vi "_kafkaEventsToWaveform - Copy.vi"(8 "error":errorcluster, 10 "Waveform Datatype":variant, 11 "Kafka Events":T1[](array[typedef])) -> (0 "error out":errorcluster, 3 "Waveforms":waveform(dbl)[](array[waveform]), 5 "Names":string[][](array[string]), 7 "Values":variant[][](array[variant]))   [LabVIEW 2019]
uses:
  KafkaLVLib/API/KafkaConsumerEvent.ctl
  b523245a-1091-4a37-a3a5-079169cc6668.vi
  54bb518a-e9be-4d14-b53e-b2dc3388e6d5.vi
  fe8c1a35-af5e-47a5-bbcb-22ec2aeec76b.vi
  <vilib>/JDP Science/JSONtext/String Subset.vi
  <vilib>/JDP Science/JSONtext/Parsing/Parse Full Path or Item Name.vi
  <vilib>/JDP Science/JSONtext/Next JSON Value.vi
  <vilib>/JDP Science/JSONtext/support/Error Cluster From Code.vi
  <vilib>/JDP Science/JSONtext/Offset/Find Item Locations by Path.vi
  <vilib>/JDP Science/JSONtext/JSON text to Variant.vi
  <vilib>/JDP Science/JSONtext/JSONtext.lvlib
panel:
  out "Measured Data":waveform(dbl)[](graph)
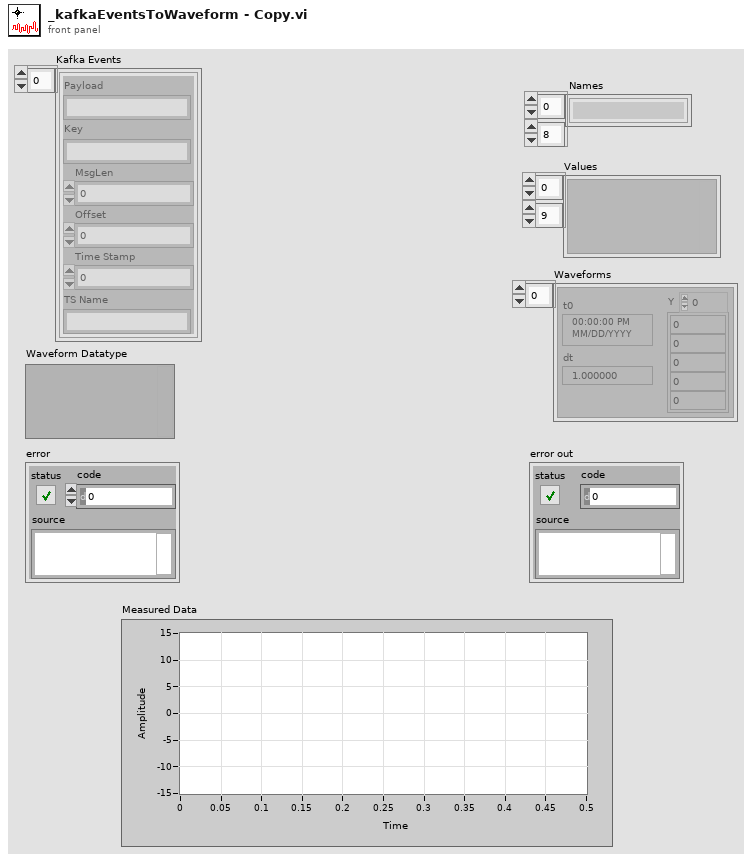
[diagram p1: front panel]
types:
  T1 = typedef "KafkaConsumerEvent.ctl" = cluster{"Payload":string, "Key":string, "MsgLen":u64, "Offset":i64, "Time Stamp":i64, "TS Name":string}
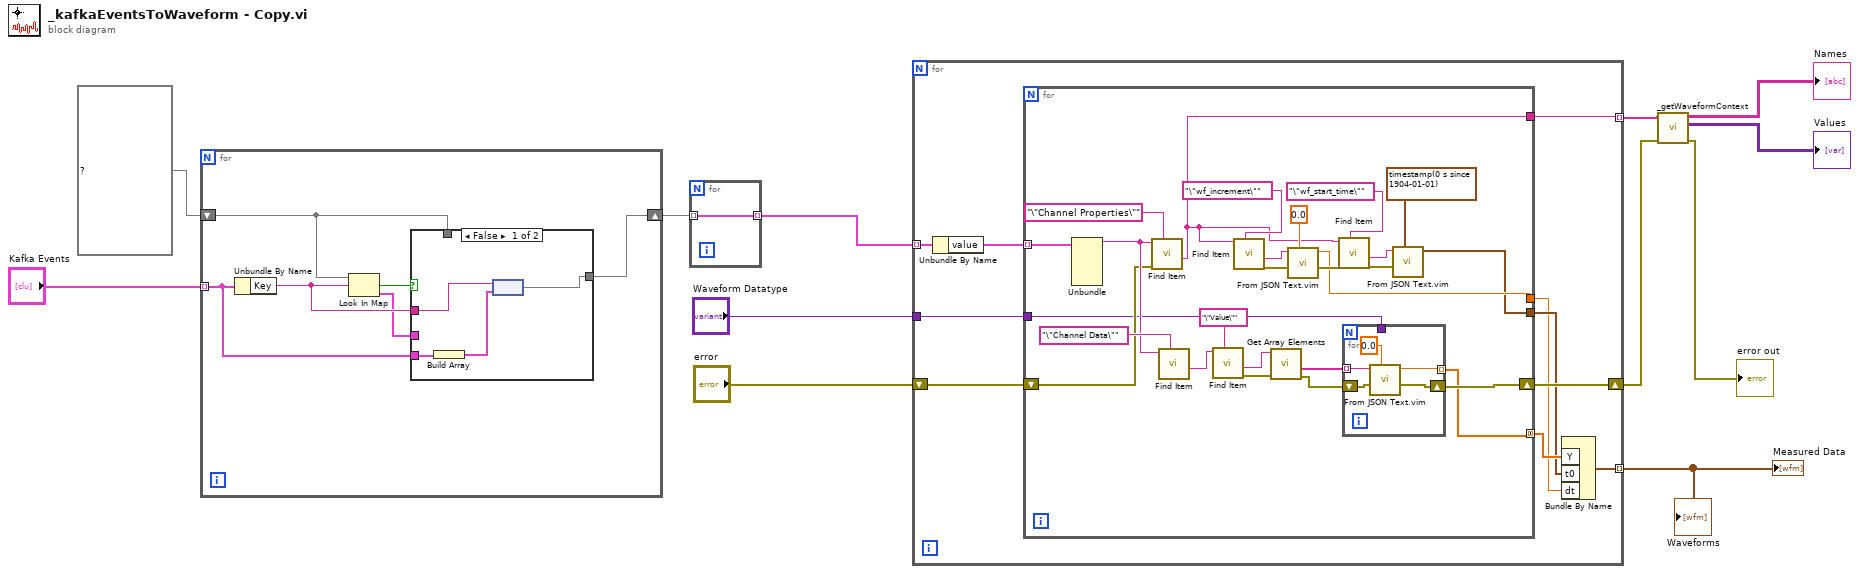
[diagram p0: block diagram]
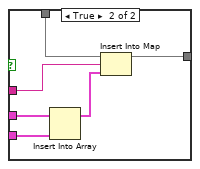
[diagram p2: hidden frame]
diagram:
  n1 = for {
    tunnel: "Kafka Events" -> [w13] mode=indexing
    shift-right: [w16] -> w4
    shift-left: map{string, T1[]} {} ("map") -> [w17]
    n2 = Unbundle By Name(w13) -> ("Key"=w15:string)
    n3 = Look In Map(map=w17, key=w15) -> (key not found?=w18:bool, value=w14:T1[])  [unwired: 1 in]
    n4 = case shown="False" w18 {
      tunnel: w17 -> [_ w28]
      tunnel: [w19 w27] -> w16
      tunnel: w15 -> [w22 w26]
      tunnel: w14 -> [_ w25]
      tunnel: w13 -> [w21 w24]
      frame False {
        n5 = Build Array(w21) -> (w20:T1[])
        n6 = node(w22, w20) -> (w19:map{string, T1[]})
      }
      frame True {
        n7 = Insert Into Array(array=w25, new element=w24) -> (w23:T1[])  [unwired: 1 in]
        n8 = Insert Into Map(map in=w28, key=w26, value=w23) -> (map out=w27:map{string, T1[]})  [unwired: 2 out]
      }
    }
  }
  n9 = for {
    tunnel: [w29] -> w1 mode=indexing
    tunnel: w4 -> [w29] mode=indexing
  }
  n10 = for {
    tunnel: w1 -> [w39] mode=indexing
    shift-right: [w36] -> w8
    shift-left: "error" -> [w37]
    tunnel: [w35] -> w11 mode=indexing
    tunnel: [w31] -> w9 mode=indexing
    tunnel: "Waveform Datatype" -> [w30]
    n11 = Unbundle By Name(w39) -> ("value"=w38:T1[])
    n12 = for {
      tunnel: w38 -> [w65] mode=indexing
      shift-right: [w54] -> w36
      shift-left: w37 -> [w55]
      tunnel: [w44] -> w32
      tunnel: [w43] -> w33
      tunnel: [w42] -> w34 mode=concatenating
      tunnel: [w41] -> w31
      tunnel: w30 -> [w40]
      n13 = Unbundle(w65) -> ("Payload"=w62:string)  [unwired: 5 out]
      n14 = call <vilib>:"Find Item.vi"("$Path or Item Name"="\"Channel Properties\"", "error in (no error)"=w55, "JSON"=w62) -> ("<JSON>"=w41:string)  [unwired: 5 in, 3 out]
      n15 = call <vilib>:"Find Item.vi"("$Path or Item Name"="\"Channel Data\"", "JSON"=w62) -> ("<JSON>"=w61:string)  [unwired: 6 in, 3 out]
      n16 = call <vilib>:"Find Item.vi"("$Path or Item Name"="\"Value\"", "JSON"=w61) -> ("error out"=w59:errorcluster, "<JSON>"=w58:string)  [unwired: 6 in, 2 out]
      n17 = call <vilib>:"Find Item.vi"("$Path or Item Name"="\"wf_increment\"", "JSON"=w41) -> ("error out"=w52:errorcluster, "<JSON>"=w53:string)  [unwired: 6 in, 2 out]
      n18 = call <vilib>:"Get Array Elements.vi"("error in (no error)"=w59, "JSON"=w58) -> ("error out"=w56:errorcluster, "<JSON>"=w57:string[])  [unwired: 7 in, 1 out]
      n19 = call "From JSON Text.vim"("Data Type and Default Value"=0.0, "error in (no error)"=w52, "JSON"=w53) -> ("error out"=w49:errorcluster, "Data out"=w44:dbl)  [unwired: 7 in]
      n20 = call <vilib>:"Find Item.vi"("$Path or Item Name"="\"wf_start_time\"", "error in (no error)"=w49, "JSON"=w41) -> ("error out"=w51:errorcluster, "<JSON>"=w50:string)  [unwired: 5 in, 2 out]
      n21 = for {
        tunnel: w57 -> [w70] mode=indexing
        shift-right: [w67] -> w54
        shift-left: w56 -> [w69]
        tunnel: [w68] -> w42 mode=indexing
        tunnel: w40 -> [_]
        n22 = call "From JSON Text.vim"("Data Type and Default Value"=0.0, "error in (no error)"=w69, "JSON"=w70) -> ("error out"=w67:errorcluster, "Data out"=w68:dbl)  [unwired: 7 in]
      }
      n23 = call "From JSON Text.vim"("Data Type and Default Value"=timestamp(0 s since 1904-01-01) ("t0"), "error in (no error)"=w51, "JSON"=w50) -> ("Data out"=w43:timestamp)  [unwired: 7 in, 1 out]
    }
    n24 = Bundle By Name("Y"=w34, "t0"=w33, "dt"=w32) -> (w35:waveform(dbl))  [unwired: 1 in]
  }
  "Measured Data" <- w11
  "Waveforms" <- w11
  n25 = call "_getWaveformContext.vi"("error in"=w8, "Context"=w9) -> ("error out"=→"error out":errorcluster, "Values"=→"Values":variant[][], "Names"=→"Names":string[][])  [unwired: 7 in]
